vi "Get IFW Register Clock.vi"(2 "reference fpga":refnum<class "niUSRP Reference FPGA v1.lvclass">) -> (4 "ifw register clock":refnum<k21>)   [LabVIEW 2025, in "niUSRP Reference FPGA v1.lvclass"]
uses:
  niUSRP Reference FPGA v1.lvclass
  niUSRP Reference FPGA v1.lvclass/niUSRP Reference FPGA v1.ctl
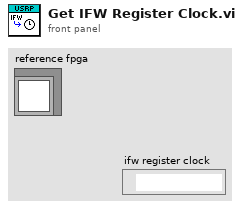
[diagram p1: front panel]
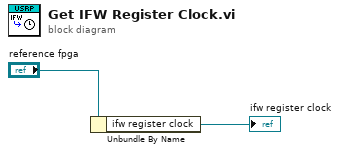
[diagram p0: block diagram]
diagram:
  n1 = Unbundle By Name("reference fpga") -> ("ifw register clock"=→"ifw register clock":refnum<k21>)
